vi "dispose server acceptor.vi"(8 "error in":errorcluster, 11 "server acceptor in":refnum<class "server acceptor.lvclass">) -> (0 "error out":errorcluster)   [LabVIEW 2016, in "server acceptor.lvclass"]
uses:
  server acceptor.lvclass
  C:/Users/IEUser/Desktop/libasynclvtls/tls classes/connection creator/connection creator.lvclass
  server acceptor.lvclass/server acceptor.ctl
  dllwrapper/library path.vi
  <vilib>/Utility/error.llb/Error Cluster From Error Code.vi
  connection creator.lvclass
  dllwrapper/async tls dl.lvlib
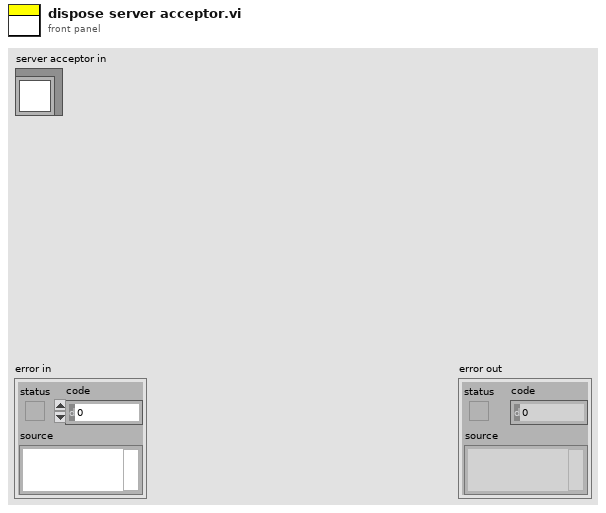
[diagram p1: front panel]
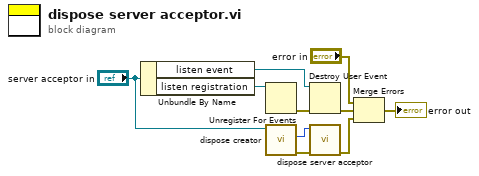
[diagram p0: block diagram]
diagram:
  n1 = Unbundle By Name("server acceptor in") -> ("listen event"=w3:refnum<user-event>, "listen registration"=w2:refnum<event-registration>)
  n2 = Unregister For Events(event registration refnum=w2) -> (error out=w4:errorcluster)  [unwired: 1 in]
  n3 = call "dispose creator.vi"("connection creator in"="server acceptor in") -> ("error out"=w7:errorcluster, "pointer"=w6:u64)  [unwired: 9 in]
  n4 = Destroy User Event(user event=w3, error in=w4) -> (error out=w1:errorcluster)
  n5 = call "dispose server acceptor.vi"("error in"=w7, "acceptor"=w6) -> ("error out"=w8:errorcluster)  [unwired: 9 in]
  n6 = Merge Errors("error in", w1, w8) -> (→"error out":errorcluster)
